vi "hmi_browse_folder.vi"(7 "description":string, 8 "error in (no error)":errorcluster, 11 "folder":string) -> (0 "error out":errorcluster, 3 "selected path":path)   [LabVIEW 2015, in "lv-builder-default.lvlib"]
uses:
  lv-builder-default.lvlib
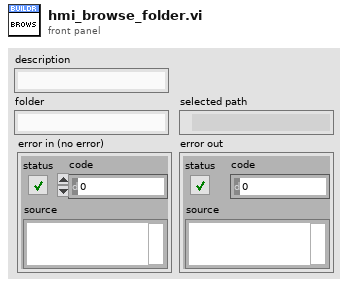
[diagram p1: front panel]
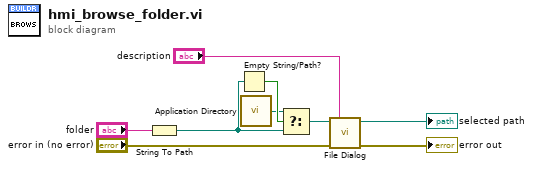
[diagram p0: block diagram]
diagram:
  n1 = String To Path(string="folder") -> (path=w1:path)
  n2 = Empty String/Path?(string/path=w1) -> (empty?=w6:bool)
  n3 = call <vilib>:"Application Directory.vi"() -> ("Application Directory"=w4:path)
  n4 = Select(t=w4, s=w6, f=w1) -> (s? t:f=w7:path)
  n5 = call "File Dialog"("start path"=w7, "prompt"="description", "error in"="error in (no error)") -> ("selected path"=→"selected path":path, "error out"=→"error out":errorcluster)  [unwired: 9 in, 2 out]
